vi "Conditional Quit LabVIEW.vi"(8 "error in (no error)":errorcluster) -> (0 "error out":errorcluster)   [LabVIEW 2017]
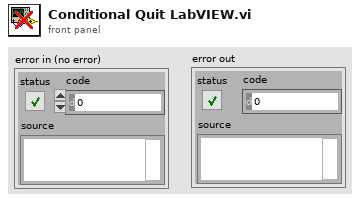
[diagram p1: front panel]
types:
  T1 = enum32{"invalid app kind", "Development System", "Run Time System", "Student Edition", "Embedded LabVIEW", "Evaluation", "Custom"}
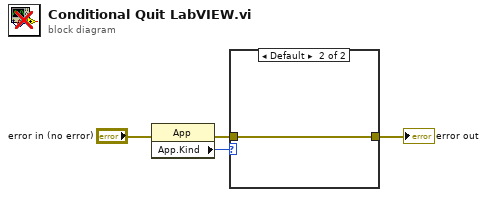
[diagram p0: block diagram]
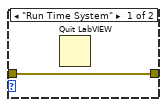
[diagram p2: hidden frame]
diagram:
  n1 = property class="App"(error in="error in (no error)") -> (error out=w1:errorcluster, "App.Kind"=w4:T1)  [unwired: 1 in, 1 out]
  n2 = case shown="Default" w4 {
    tunnel: w1 -> [w5 w6]
    tunnel: [w5 w6] -> w2
    frame "Run Time System" {
      n3 = Quit LabVIEW() -> ()  [unwired: 1 in]
    }
    frame Default {
    }
  }
  "error out" <- w2
